vi "Find Red Pitaya Digitizers.vi"(6 "Timeout":i32=100, 7 "Logic tags":u16[](array[numeric])=[101, 102, 104, 107, 108, 109, 111], 8 "Error In":errorcluster, 9 "End address":i32=120, 10 "Start address":i32=100, 11 "Subnet":string="192.168.1") -> (0 "Error Out":errorcluster, 1 "Addresses":string[](array[string]), 2 "Device names":string[](array[string]), 3 "Digitizers out":refnum<class "Red Pitaya Digitizer.lvclass">[](array[class]))   [LabVIEW 2016]
uses:
  Red Pitaya Digitizer.lvclass
  C:/github/NHMFL_Core/Libraries/Instruments/Instrument Driver/Instrument Driver.lvclass
  RP Core/Rep Pitaya I-V driver/RP I-V Driver.lvclass
  C:/github/NHMFL_Core/Libraries/Red Pitaya/Red Pitaya Digitizer/Red Pitaya Digitizer.lvclass
  Red Pitaya Digitizer.lvclass/Red Pitaya Digitizer.ctl
  Instruments/Instrument Driver/Instrument Driver.lvclass/Instrument Driver.ctl
  RP Core/RP Instrument/RP Instrument.lvclass/RP Instrument.ctl
  Write Logic tag.vi
  Read RP Instrument.vi
  Instruments/Instrument Driver/Write Type ID.vi
  RP Core/RP Instrument/Write Samples per trigger increment .vi
  RP Core/RP Instrument/Write bytes per sample.vi
  Write RP Instrument.vi
  Write Server address.vi
  RP Core/RP Instrument/RP Instrument.lvclass
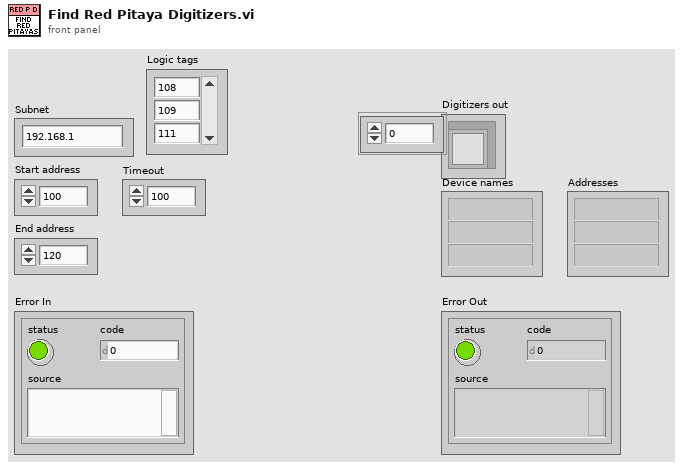
[diagram p1: front panel]
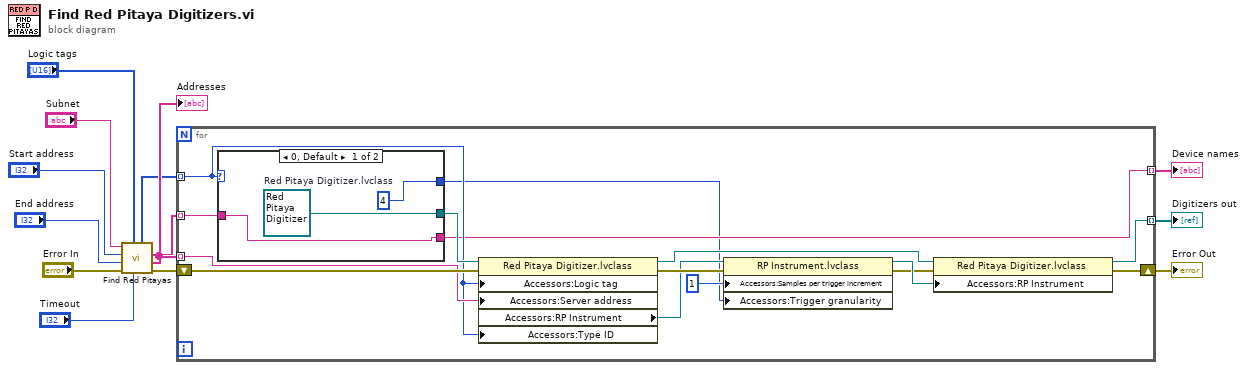
[diagram p0: block diagram]
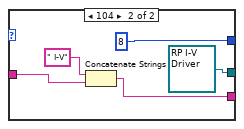
[diagram p2: hidden frame]
diagram:
  n1 = call "Find Red Pitayas.vi"("Timeout"="Timeout", "Acceptable logic tags"="Logic tags", "Error In"="Error In", "End address"="End address", "Start address"="Start address", "Subnet"="Subnet") -> ("Error Out"=w5:errorcluster, "Addresses"=w7:string[], "Device names"=w2:string[], "Logic tags out"=w3:u16[])  [unwired: 2 in]
  "Addresses" <- w7
  n2 = for {
    tunnel: w7 -> [w18] mode=indexing
    shift-right: [w23] -> w13
    shift-left: w5 -> [w27]
    tunnel: [w19] -> w12 mode=indexing
    tunnel: w3 -> [w17] mode=indexing
    tunnel: w2 -> [w16] mode=indexing
    tunnel: [w15] -> w1 mode=indexing
    n3 = case shown="0, Default" w17 {
      tunnel: [w31 refnum<class "RP I-V Driver.lvclass"> refnum ("RP I-V Driver.lvclass")] -> w28
      tunnel: w16 -> [w30 w33]
      tunnel: [w30 w35] -> w15
      tunnel: [4 ("Trigger granularity") 8 ("Trigger granularity")] -> w14
      frame 0, Default {
        w31 = refnum<class "Red Pitaya Digitizer.lvclass"> refnum  # Red Pitaya Digitizer.lvclass
      }
      frame 104 {
        n4 = Concatenate Strings(" I-V" ("string"), w33) -> (w35:string)
      }
    }
    n5 = property class="Red Pitaya Digitizer.lvclass"(reference=w28, error in=w27, "Accessors:Logic tag"=w17, "Accessors:Server address"=w18, "Accessors:Type ID"=w17) -> (reference out=w20:refnum<class "Red Pitaya Digitizer.lvclass">, error out=w26:errorcluster, "Accessors:RP Instrument"=w25:refnum<class "RP Instrument.lvclass">)
    n6 = property class="RP Instrument.lvclass"(reference=w25, error in=w26, "Accessors:Samples per trigger increment "=1 ("Samples per trigger increment"), "Accessors:Trigger granularity"=w14) -> (reference out=w22:refnum<class "RP Instrument.lvclass">, error out=w21:errorcluster)
    n7 = property class="Red Pitaya Digitizer.lvclass"(reference=w20, error in=w21, "Accessors:RP Instrument"=w22) -> (reference out=w19:refnum<class "Red Pitaya Digitizer.lvclass">, error out=w23:errorcluster)
  }
  "Digitizers out" <- w12
  "Device names" <- w1
  "Error Out" <- w13
